vi "Shutdown.vi"(8 "error in (no error)":errorcluster, 11 "ATS9350 in":refnum<class "ATS9350.lvclass">) -> (0 "error out":errorcluster, 3 "ATS9350 out":refnum<class "ATS9350.lvclass">)   [LabVIEW 2015, in "ATS9350.lvclass"]
uses:
  ATS9350.lvclass
  ATS-VI/ATS_ctl/ATS_Async_Ctrl.ctl
  DAQ Class.lvclass
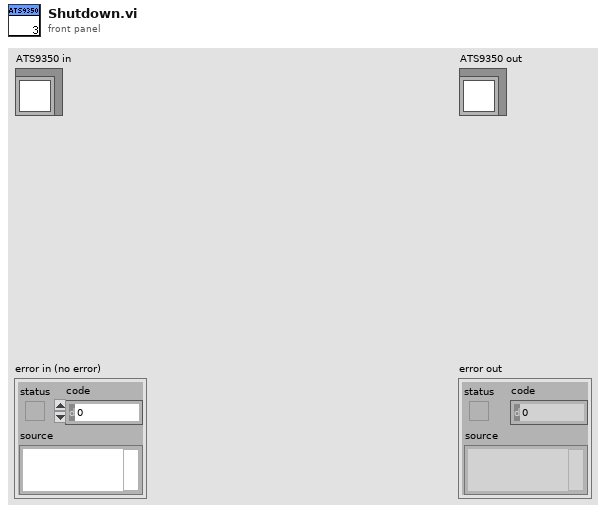
[diagram p1: front panel]
types:
  T1 = typedef "ATS_Async_Ctrl.ctl" = enum16{"SetupDMA", "StartCapture", "Get", "Get_Stream", "Abort", "Stop"}
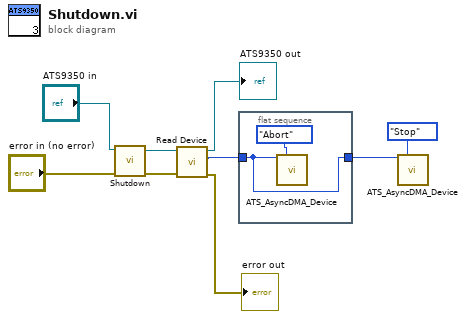
[diagram p0: block diagram]
diagram:
  n1 = call-parent "Shutdown.vi"("error in (no error)"="error in (no error)", "DAQ Class in"="ATS9350 in") -> ("error out"=w4:errorcluster, "DAQ Class out"=w3:refnum<class "ATS9350.lvclass">)  [unwired: 8 in]
  n2 = call-dynamic "Read Device.vi"("error in (no error)"=w4, "ATS9350 in"=w3) -> ("error out"=→"error out":errorcluster, "Device"=w7:i32, "ATS9350 out"=→"ATS9350 out":refnum<class "ATS9350.lvclass">)  [unwired: 7 in]
  n3 = flat-sequence {
    tunnel: w7 -> [w10]
    tunnel: [w10] -> w6
    frame #0 {
      n4 = call "ATS_AsyncDMA_Device.vi"("DeviceIn"=w10, "ATS_Async_Ctrl"=ATS_Async_Ctrl."Abort") -> ()  [unwired: 9 in, 5 out]
    }
  }
  n5 = call "ATS_AsyncDMA_Device.vi"("DeviceIn"=w6, "ATS_Async_Ctrl"=ATS_Async_Ctrl."Stop") -> ()  [unwired: 9 in, 5 out]
